vi "Result_Test.vi"(8 "error in (no error)":errorcluster caption="entrée d'erreur (pas d'erreur)", 11 "Flash_Jlink en entrée":refnum<class "Check_Type.lvclass">) -> (0 "error out":errorcluster caption="sortie d'erreur", 3 "Flash_Jlink en sortie":refnum<class "Check_Type.lvclass">)   [LabVIEW 2020, in "Library Test.lvlib" / "Check_Type.lvclass"]
uses:
  Check_Type.lvclass
  C:/Users/ngarcin/OneDrive - Altyor/Standard TB/Suite TB45/Class/Test/Test (Default)/Test (Default).lvclass
  Commun VI/TypeDef/Variable Printable.ctl
  Test_Without_Instr/Test_Without_Inst.lvclass
  Commun VI/Library Commun.lvlib
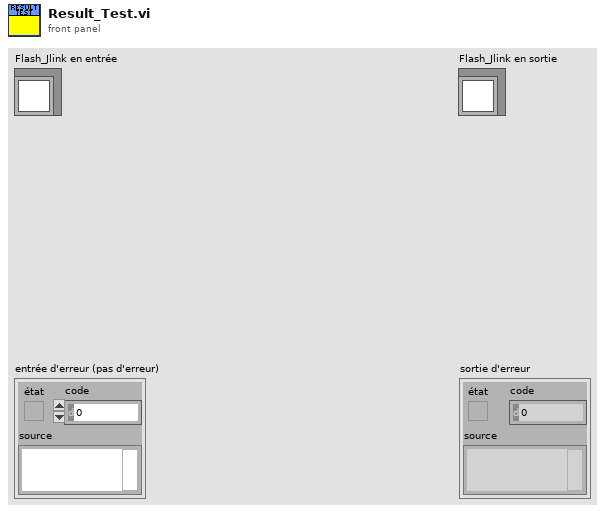
[diagram p1: front panel]
types:
  T1 = enum16{"Get Variable", "Get All Variables", "Set Variable", "Delete Variable", "Delete All Variable"}
  T2 = typedef "Variable Printable.ctl" = string
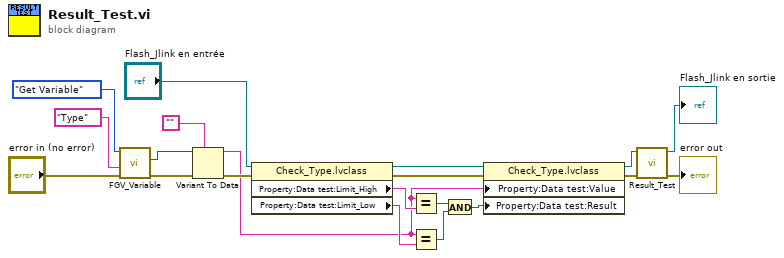
[diagram p0: block diagram]
diagram:
  n1 = call "FGV_Variable.vi"("error in (no error)"="error in (no error)", "Variable"=T2 "Type", "Function"=T1."Get Variable") -> ("error out"=w15:errorcluster, "Data Out"=w14:variant)  [unwired: 6 in, 1 out]
  n2 = Variant To Data(error in=w15, type="", Variant=w14) -> (data=w1:string, error out=w6:errorcluster)
  n3 = property class="Check_Type.lvclass"(reference="Flash_Jlink en entrée", error in=w6) -> (reference out=w3:refnum<class "Check_Type.lvclass">, error out=w12:errorcluster, "Property:Data test:Limit_High"=w11:string, "Property:Data test:Limit_Low"=w10:string)
  n4 = Equal?(x=w1, y=w11) -> (x = y?=w9:bool)
  n5 = Equal?(x=w1, y=w10) -> (x = y?=w8:bool)
  n6 = And(x=w9, y=w8) -> (x .and. y?=w7:bool)
  n7 = property class="Check_Type.lvclass"(reference=w3, error in=w12, "Property:Data test:Value"=w1, "Property:Data test:Result"=w7) -> (reference out=w4:refnum<class "Check_Type.lvclass">, error out=w5:errorcluster)
  n8 = call-parent "Result_Test.vi"("error in (no error)"=w5, "Test_Without_Inst en entrée"=w4) -> ("error out"=→"error out":errorcluster, "Test_Without_Inst en sortie"=→"Flash_Jlink en sortie":refnum<class "Check_Type.lvclass">)  [unwired: 8 in]
